vi "Vision Processing Ian.vi"(4 "error in (no error)":errorcluster, 7 "Image Size Gear":T4=enum."160x120") -> ()   [LabVIEW 2016]
doc: "This VI runs in parallel to other tasks. It gets images from the camera, processes them for color or shape and use that information to affect robot behavior."
uses:
  Vision Support Code/Camera Types.ctl
  <vilib>/Rock Robotics/WPI/Camera/WPI_CameraImageSize.ctl
  <vilib>/vision/Measure.llb/Edge Options.ctl
  <vilib>/vision/Measure.llb/Edge Polarity.ctl
  <vilib>/Rock Robotics/WPI/Camera/WPI_CameraExposure Values.ctl
  <vilib>/Rock Robotics/WPI/Camera/WPI_CameraWhite Balance Values.ctl
  <vilib>/Rock Robotics/WPI/Camera/WPI_CameraFrameRate.ctl
  <vilib>/vision/NI_Vision_Development_Module.lvlib
panel:
  in  "Edge Options Gear":T1={"Edge Polarity"=0, "Kernel Size"=3, "Width"=3, "Minimum Edge Strength"=18.0, "Interpolation Type"=enum."Bilinear Fixed", "Data Processing Method"=enum."Average"} {"Edge Polarity" items=["All Edges", "Rising Edges", "Falling Edges"]; "Minimum Edge Strength" format="%.2f"; "Width" step=2; "Kernel Size" step=2}
  in  "boresight":dbl=24.9
  in  "Factor to Distance":dbl=12.0
  in  "Ball?":bool=TRUE
  in  "LED Color Ball":T3={"Hue"={189.50518161930526, 233.66474196477665}, "Sat"={33.39285714285715, 185.17857142857144}, "Val"={15.178571428571438, 255.0}} {"Hue" scale=0.0..255.0 scale format="%#_3g"}
  in  "Brightness":i32=30
  in  "Exposure (%)":dbl format="%#_13g"
  in  "Color Temp (K)":dbl=4000.0 format="%#_13g"
  in  "Edge Options":T1={"Edge Polarity"=0, "Kernel Size"=3, "Width"=3, "Minimum Edge Strength"=2.0, "Interpolation Type"=enum."Bilinear Fixed", "Data Processing Method"=enum."Average"} {"Edge Polarity" items=["All Edges", "Rising Edges", "Falling Edges"]; "Minimum Edge Strength" format="%.2f"; "Width" step=2; "Kernel Size" step=2}
  in  "Size Limit %":dbl=0.04 format="%#_13g"
  in  "Cal Turret":bool
  out "Calibration error 2":errorcluster={"status"=TRUE, "code"=-1074396074, "source"=""}
  out "Physical Paths":string[](array[string])=["-0_1_1_1_0", "-0_1_2_1_0"]
  out "Logical Paths":string[](array[string])=["video0", "video1"]
  out "Gear Valid":bool
  out "Boiler Yaw Delta":dbl=-17.15
  out "Boiler Valid":bool
  out "Boiler Distance":dbl=inf
  in  "Angle":enum16{"Horizontal", "Vertical", "Diagonal"}(ring)=enum."Vertical"
  in  "Gear?":bool=TRUE
  in  "Image SizeTurr":T4=enum."160x120"
  in  "Score Cutoff Turret":dbl=70.0
  out "Gear Distance":dbl=inf
  out "Gear Yaw Delta":dbl=-5.600000000000001
  in  "FOV":cluster{"X (degrees)":dbl, "Y (degrees)":dbl}={"X (degrees)"=34.3, "Y (degrees)"=61.0}
  in  "Height":T5={"Hc (GND to lense)"=12.5, "Ht (GND to CTR)"=0.0}
  in  "LED Color Target":T3={"Hue"={217.1650671807445, 7.296259223023774}, "Sat"={115.35714285714286, 255.0}, "Val"={21.25000000000001, 255.0}} {"Hue" scale=0.0..255.0 scale format="%#_3g"}
  in  "Camera Type":T6=enum."1013"
  in  "Score Cutoff %":dbl=50.0
  in  "Particles":dbl=5.0
  in  "Color Mode":u16(ring)=3 items=["RGB", "HSL", "HSV", "HSI"]
  in  "Use Calibration":bool
  out "Calibration error":errorcluster
  in  "Line Border":cluster{"Top":dbl, "Bottom":dbl}={"Top"=6.0, "Bottom"=1.0}
  in  "Display Original":bool=TRUE
  in  "Display Mask":bool=TRUE
  out "Mask":T7(plugin-control)
  out "Original Image":T7(plugin-control)
  out "loop ms":u32=117
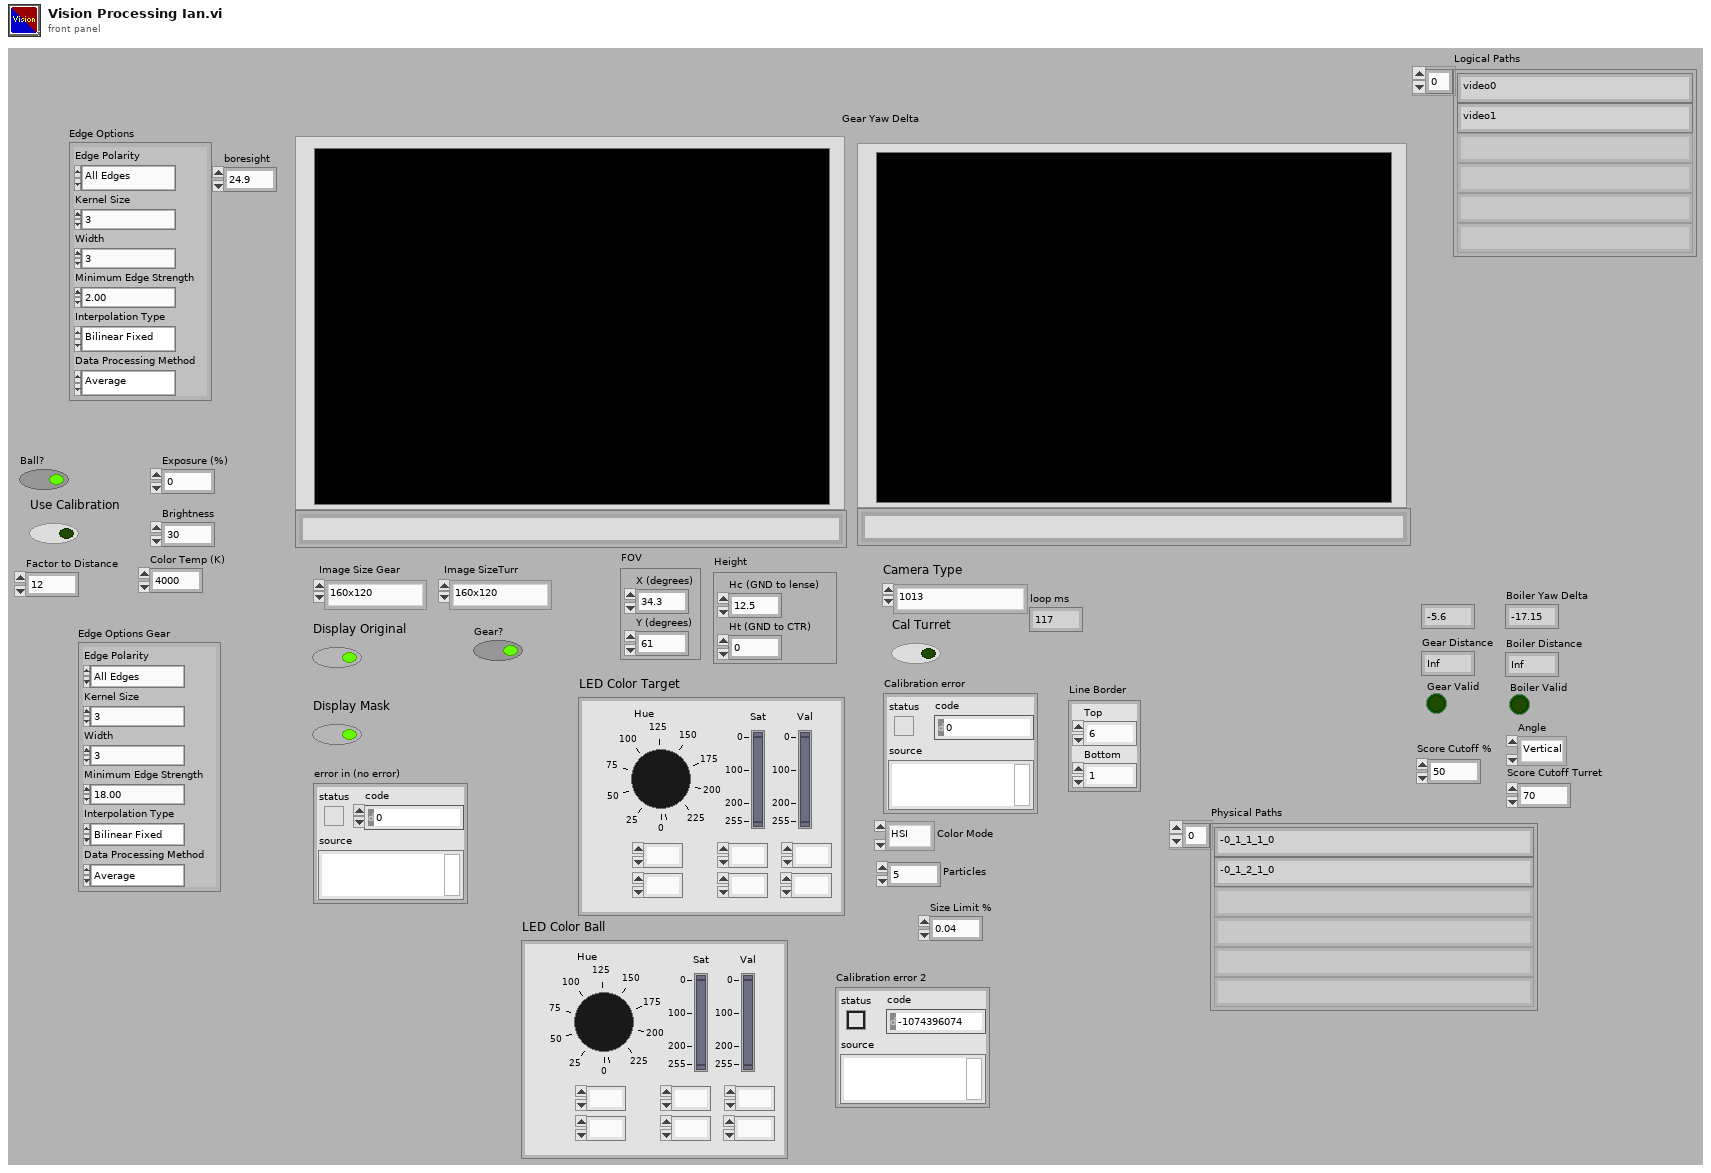
[diagram p1: front panel]
types:
  T1 = typedef "Edge Options.ctl" = cluster{"Edge Polarity":T2, "Kernel Size":u32, "Width":u32, "Minimum Edge Strength":sgl, "Interpolation Type":enum32{"Zero Order", "Bilinear", "Quadratic", "Cubic", "Bilinear Fixed"}, "Data Processing Method":enum32{"Average", "Median"}}
  T2 = typedef "Edge Polarity.ctl" = u32
  T3 = cluster{"Hue":cluster{dbl, dbl}, "Sat":cluster{dbl, dbl}, "Val":cluster{dbl, dbl}}
  T4 = typedef "WPI_CameraImageSize.ctl" = enum16{"640x480", "320x240", "160x120", "Custom"}
  T5 = cluster{"Hc (GND to lense)":dbl, "Ht (GND to CTR)":dbl}
  T6 = typedef "Camera Types.ctl" = enum16{"206", "1011", "1013", "MS HD3000 square", "MS HD3000 640x480"}
  T7 = typedef "IMAQ Image.ctl" = refnum<image>
  T8 = typedef "Image Type" = u32
  T9 = typedef "WPI_CameraFrameRate.ctl" = u32
  T10 = typedef "WPI_CameraExposure Values.ctl" = enum16{"Auto", "Flicker-free 50 Hz", "Flicker-free 60 Hz", "Hold current", "Custom"}
  T11 = typedef "WPI_CameraWhite Balance Values.ctl" = enum16{"Auto", "Fixed indoor", "Fixed outdoor 1", "Fixed outdoor 2", "Fixed fluorescent 1", "Fixed fluorescent 2", "Hold current", "Custom"}
  T12 = typedef "Particle Parameters" = i32
  T13 = typedef "WPI_CameraDevRef.ctl" = cluster{"Camera Address":string, "CameraStatus":errorcluster}
  T14 = cluster{"Left":dbl, "Top":dbl, "Right":dbl, "Bottom":dbl}
  T15 = cluster{"Distance (ft)":dbl, "Score":dbl, "Normalized":cluster{"Center":cluster{dbl, dbl}, "Rectangle":cluster{"Numeric":dbl, "Numeric 2":dbl, "Numeric 3":dbl, "Numeric 5":dbl}}, "Pixels":cluster{"Center":cluster{dbl, dbl}, "Rectangle":cluster{"Numeric":dbl, "Numeric 2":dbl, "Numeric 3":dbl, "Numeric 5":dbl}}}
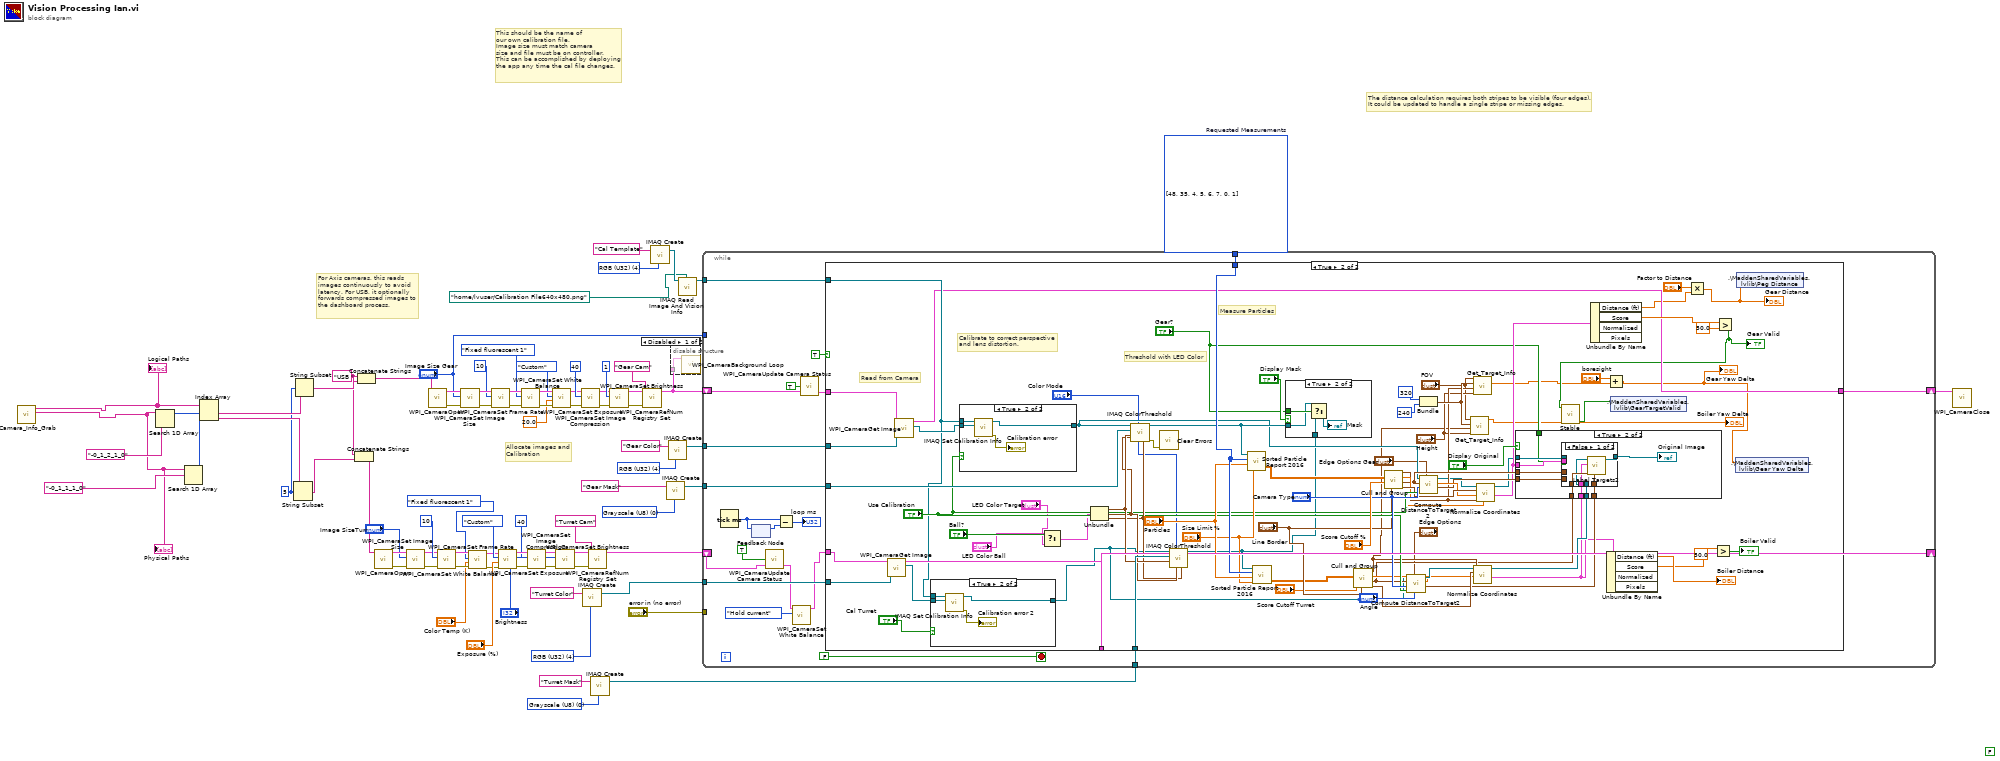
[diagram p0: block diagram]
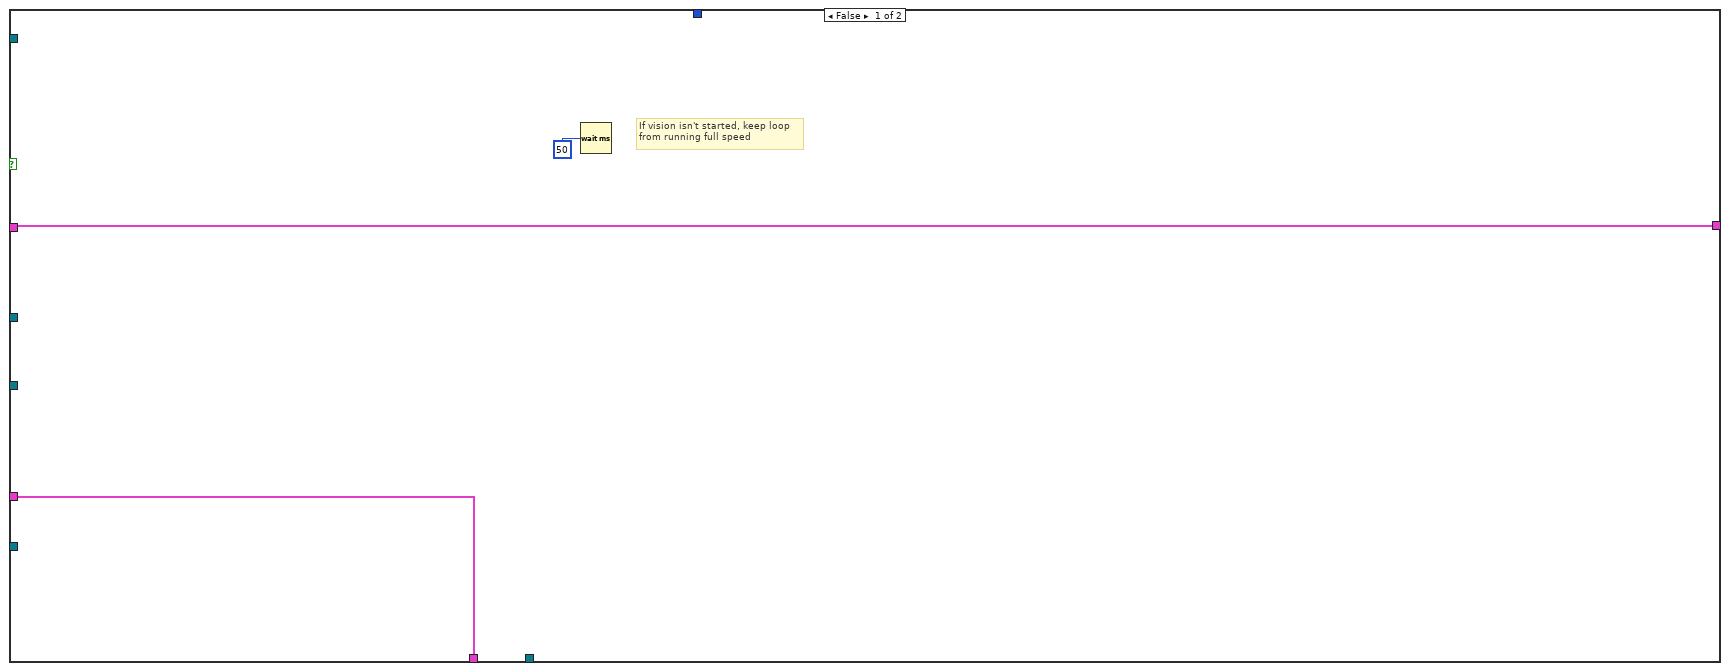
[diagram p3: hidden frame]
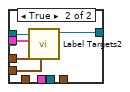
[diagram p6: hidden frame]
diagram:
  (unwired) FALSE
  w14 = "USB " ("string")
  w16 = 5 ("offset (0)")
  w24 = T8 0 items=["Grayscale (U8)", "Grayscale (I16)", "Grayscale (SGL)", "Complex (CSG)", "RGB (U32)", "HSL (U32)", "RGB (U64)", "Grayscale (U16)"] ("Image Type")
  w26 = T8 4 items=["Grayscale (U8)", "Grayscale (I16)", "Grayscale (SGL)", "Complex (CSG)", "RGB (U32)", "HSL (U32)", "RGB (U64)", "Grayscale (U16)"] ("Image Type")
  w74 = T8 4 items=["Grayscale (U8)", "Grayscale (I16)", "Grayscale (SGL)", "Complex (CSG)", "RGB (U32)", "HSL (U32)", "RGB (U64)", "Grayscale (U16)"] ("Image Type")
  w79 = T8 0 items=["Grayscale (U8)", "Grayscale (I16)", "Grayscale (SGL)", "Complex (CSG)", "RGB (U32)", "HSL (U32)", "RGB (U64)", "Grayscale (U16)"] ("Image Type")
  w80 = T8 4 items=["Grayscale (U8)", "Grayscale (I16)", "Grayscale (SGL)", "Complex (CSG)", "RGB (U32)", "HSL (U32)", "RGB (U64)", "Grayscale (U16)"] ("Image Type")
  w76 = T12[] [48, 35, 4, 5, 6, 7, 0, 1] items=["Center of Mass X", "Center of Mass Y", "First Pixel X", "First Pixel Y", "Bounding Rect Left", "Bounding Rect Top", "Bounding Rect Right", "Bounding Rect Bottom", "Max Feret Diameter Start X", "Max Feret Diameter Start Y", "Max Feret Diameter End X", "Max Feret Diameter End Y", "Max Horiz. Segment Length Left", "Max Horiz. Segment Length Right", "Max Horiz. Segment Length Row", "-", "Bounding Rect Width", "Bounding Rect Height", "Bounding Rect Diagonal", "Perimeter", "Convex Hull Perimeter", "Holes' Perimeter", "Max Feret Diameter", "Equivalent Ellipse Major Axis", "Equivalent Ellipse Minor Axis", "Equivalent Ellipse Minor Axis (Feret)", "Equivalent Rect Long Side", "Equivalent Rect Short Side", "Equivalent Rect Diagonal", "Equivalent Rect Short Side (Feret)", "Average Horiz. Segment Length", "Average Vert. Segment Length", "Hydraulic Radius", "Waddel Disk Diameter", "-", "Area", "Holes' Area", "Particle & Holes' Area", "Convex Hull Area", "Image Area", "-", "Number of Holes", "Number of Horiz. Segments", "Number of Vert. Segments", "-", "Orientation", "Max Feret Diameter Orientation", "-", "% Area/Image Area", "% Area/(Particle & Holes' Area)", "Ratio of Equivalent Ellipse Axes", "Ratio of Equivalent Rect Sides", "-", "Elongation Factor", "Compactness Factor", "Heywood Circularity Factor", "Type Factor", "-", "Sum X", "Sum Y", "Sum XX", "Sum XY", "Sum YY", "Sum XXX", "Sum XXY", "Sum XYY", "Sum YYY", "-", "Moment of Inertia XX", "Moment of Inertia XY", "Moment of Inertia YY", "Moment of Inertia XXX", "Moment of Inertia XXY", "Moment of Inertia XYY", "Moment of Inertia YYY", "Norm. Moment of Inertia XX", "Norm. Moment of Inertia XY", "Norm. Moment of Inertia YY", "Norm. Moment of Inertia XXX", "Norm. Moment of Inertia XXY", "Norm. Moment of Inertia XYY", "Norm. Moment of Inertia YYY", "Hu Moment 1", "Hu Moment 2", "Hu Moment 3", "Hu Moment 4", "Hu Moment 5", "Hu Moment 6", "Hu Moment 7"]  # Requested Measurements
  # "For Axis cameras, this reads\nimages continuously to avoid\nlatency. For USB, it optionally\nforwards compressed images to\nthe dashboard process."
  # "Allocate images and\nCalibration"
  # "This should be the name of \nour own calibration file.\nImage size must match camera\nsize and file must be on controller.\nThis can be accomplished by deploying\nthe app any time the cal file changes."
  # "The distance calculation requires both stripes to be visible (four edges).\nIt could be updated to handle a single stripe or missing edges."
  n1 = call <userlib>:"Camera_Info_Grab.vi"() -> ("Physical Paths"=w8:string[], "Logical Paths"=w9:string[])  [unwired: 10 in]
  "Logical Paths" <- w9
  "Physical Paths" <- w8
  n2 = Search 1D Array(1D array=w8, element="-0_1_2_1_0") -> (index of element=w20:i32)  [unwired: 1 in]
  n3 = Search 1D Array(1D array=w8, element="-0_1_1_1_0") -> (index of element=w19:i32)  [unwired: 1 in]
  n4 = Index Array(array=w9, index #1=w20, index #2=w19) -> (element #1=w18:string, element #2=w17:string)
  n5 = String Subset(string=w17, offset (0)=w16) -> (substring=w13:string)  [unwired: 1 in]
  n6 = String Subset(string=w18, offset (0)=w16) -> (substring=w15:string)  [unwired: 1 in]
  n7 = Concatenate Strings(w14, w13) -> (w12:string)
  n8 = Concatenate Strings(w14, w15) -> (w11:string)
  n9 = call <vilib>:"WPI_CameraOpen.vi"("Camera Address"=w12) -> ("error out"=w39:errorcluster, "CameraDevRef"=w38:T13)  [unwired: 1 in, 8 out]
  n10 = call <vilib>:"WPI_CameraSet Image Size.vi"("error in (no error)"=w39, "Image Size"="Image SizeTurr", "CameraDevRef"=w38) -> ("error out"=w40:errorcluster, "CameraDevRef Out"=w37:T13)  [unwired: 1 in, 6 out]
  n11 = call <vilib>:"WPI_CameraOpen.vi"("Camera Address"=w11) -> ("error out"=w60:errorcluster, "CameraDevRef"=w61:T13)  [unwired: 1 in, 8 out]
  n12 = call <vilib>:"WPI_CameraSet Frame Rate.vi"("error in (no error)"=w40, "Frame Rate (fps)"=T9 10, "CameraDevRef"=w37) -> ("error out"=w4:errorcluster, "CameraDevRef Out"=w6:T13)  [unwired: 7 out]
  n13 = call <vilib>:"WPI_CameraSet Image Size.vi"("error in (no error)"=w60, "Image Size"="Image Size Gear", "CameraDevRef"=w61) -> ("error out"=w59:errorcluster, "CameraDevRef Out"=w62:T13)  [unwired: 1 in, 6 out]
  n14 = call <vilib>:"WPI_CameraSet White Balance.vi"("error in (no error)"=w4, "Color Temp (K)"="Color Temp (K)", "White Balance"=WPI_CameraWhite_Balance_Values."Fixed fluorescent 1", "CameraDevRef"=w6) -> ("error out"=w3:errorcluster, "CameraDevRef Out"=w5:T13)  [unwired: 6 in]
  n15 = call <vilib>:"WPI_CameraSet Frame Rate.vi"("error in (no error)"=w59, "Frame Rate (fps)"=T9 10, "CameraDevRef"=w62) -> ("error out"=w58:errorcluster, "CameraDevRef Out"=w64:T13)  [unwired: 7 out]
  n16 = call <vilib>:"WPI_CameraSet Exposure.vi"("error in (no error)"=w3, "Exposure (%)"="Exposure (%)", "Exposure"=WPI_CameraExposure_Values."Custom", "CameraDevRef"=w5) -> ("error out"=w41:errorcluster, "CameraDevRef Out"=w35:T13)  [unwired: 6 out]
  n17 = call <vilib>:"WPI_CameraSet White Balance.vi"("error in (no error)"=w58, "White Balance"=WPI_CameraWhite_Balance_Values."Fixed fluorescent 1", "CameraDevRef"=w64) -> ("error out"=w57:errorcluster, "CameraDevRef Out"=w63:T13)  [unwired: 1 in, 6 out]
  n18 = call <vilib>:"WPI_CameraSet Image Compression.vi"("error in (no error)"=w41, "Compression"=40, "CameraDevRef"=w35) -> ("error out"=w42:errorcluster, "CameraDevRef Out"=w36:T13)  [unwired: 7 out]
  n19 = call <vilib>:"WPI_CameraSet Exposure.vi"("error in (no error)"=w57, "Exposure (%)"=20.0, "Exposure"=WPI_CameraExposure_Values."Custom", "CameraDevRef"=w63) -> ("error out"=w56:errorcluster, "CameraDevRef Out"=w66:T13)  [unwired: 6 out]
  n20 = call <vilib>:"WPI_CameraSet Brightness.vi"("error in (no error)"=w42, "Brightness"="Brightness", "CameraDevRef"=w36) -> ("error out"=w43:errorcluster, "CameraDevRef Out"=w30:T13)  [unwired: 7 out]
  n21 = call <vilib>:"WPI_CameraSet Image Compression.vi"("error in (no error)"=w56, "Compression"=40, "CameraDevRef"=w66) -> ("error out"=w55:errorcluster, "CameraDevRef Out"=w65:T13)  [unwired: 7 out]
  n22 = call "IMAQ Create"("Image Name"="Turret Color", "Image Type"=w26) -> ("New Image"=w25:T7)  [unwired: 2 in, 2 out]
  n23 = call <vilib>:"WPI_CameraRefNum Registry Set.vi"("error in (no error)"=w43, "refnum name"="Turret Cam", "CameraDevRef"=w30) -> ("CameraDevRef"=w28:T13)  [unwired: 1 in, 7 out]
  n24 = call "IMAQ Create"("Image Name"="Turret Mask", "Image Type"=w24) -> ("New Image"=w22:T7)  [unwired: 2 in, 2 out]
  n25 = call <vilib>:"WPI_CameraSet Brightness.vi"("error in (no error)"=w55, "Brightness"=1, "CameraDevRef"=w65) -> ("error out"=w54:errorcluster, "CameraDevRef Out"=w70:T13)  [unwired: 7 out]
  n26 = call <vilib>:"WPI_CameraRefNum Registry Set.vi"("error in (no error)"=w54, "refnum name"="Gear Cam", "CameraDevRef"=w70) -> ("CameraDevRef"=w50:T13)  [unwired: 1 in, 7 out]
  n27 = call "IMAQ Create"("Image Name"="Cal Template", "Image Type"=w74) -> ("New Image"=w72:T7)  [unwired: 2 in, 2 out]
  n28 = call "IMAQ Create"("Image Name"="Gear Mask", "Image Type"=w79) -> ("New Image"=w77:T7)  [unwired: 2 in, 2 out]
  n29 = call "IMAQ Create"("Image Name"="Gear Color", "Image Type"=w80) -> ("New Image"=w75:T7)  [unwired: 2 in, 2 out]
  n30 = disable-structure shown="Disabled" {
    disable-tunnel: w50 -> [w82 _]
    frame Disabled {
      n31 = call <vilib>:"WPI_CameraBackground Loop.vi"("CameraDevRef"=w82) -> ()  [unwired: 11 in]
    }
    frame Enabled {
    }
  }
  n32 = call "IMAQ Read Image And Vision Info"("File Path"=path "/home/lvuser/Calibration File640x480.png" ("Folder Location"), "Image"=w72) -> ("Image Out"=w71:T7)  [unwired: 7 in, 2 out]
  n33 = while {
    tunnel: w75 -> [w99]
    tunnel: w77 -> [w102]
    tunnel: w76 -> [w101]
    tunnel: w71 -> [w100]
    shift-right: [w98] -> w49
    shift-left: w50 -> [w97]
    tunnel: "error in (no error)" -> [_]
    tunnel: "Image Size Gear" -> [_]
    shift-right: [w92] -> _
    shift-left: w28 -> [w87]
    tunnel: w25 -> [w91]
    tunnel: w22 -> [w90]
    stop <- FALSE ("Boolean") stop-if-true
    n34 = Tick Count (ms)() -> (millisecond timer value=w94:u32)
    n35 = feedback-in #1(w94) -> ()
    n36 = feedback #1() -> (w95:u32)  [unwired: 1 in]
    n37 = call <vilib>:"WPI_CameraUpdate Camera Status.vi"("CameraDevRef In"=w87, "Enable Vision"=TRUE) -> ("CameraDevRef Out"=w85:T13)  [unwired: 3 in]
    n38 = Subtract(x=w94, y=w95) -> (x-y=→"loop ms":u32)
    n39 = call <vilib>:"WPI_CameraSet White Balance.vi"("White Balance"=WPI_CameraWhite_Balance_Values."Hold current", "CameraDevRef"=w85) -> ("CameraDevRef Out"=w84:T13)  [unwired: 8 in, 1 out]
    n40 = call <vilib>:"WPI_CameraUpdate Camera Status.vi"("CameraDevRef In"=w97, "Enable Vision"=TRUE) -> ("CameraDevRef Out"=w96:T13)  [unwired: 3 in]
    n41 = case shown="True" TRUE {
      tunnel: w102 -> [_ w185]
      tunnel: w101 -> [_ w174]
      tunnel: w100 -> [_ w125]
      tunnel: w96 -> [w106 w184]
      tunnel: w99 -> [_ w179]
      tunnel: [w106 w120] -> w98
      tunnel: w84 -> [w104 w182]
      tunnel: [w104 w181] -> w92
      tunnel: w91 -> [_ w180]
      tunnel: w90 -> [_ w178]
      frame False {
        # "If vision isn't started, keep loop\nfrom running full speed"
        n42 = Wait (ms)(milliseconds to wait=u32 50) -> ()  [unwired: 1 out]
      }
      frame True {
        # "Read from Camera"
        # "Calibrate to correct perspective\nand lens distortion."
        # "Measure Particles"
        # "Threshold with LED Color"
        n43 = call <vilib>:"WPI_CameraGet Image.vi"("Image"=w180, "CameraDevRef"=w182) -> ("Image Out"=w124:T7, "CameraDevRef Out"=w181:T13)  [unwired: 7 in, 1 out]
        n44 = call <vilib>:"WPI_CameraGet Image.vi"("Image"=w179, "CameraDevRef"=w184) -> ("Image Out"=w137:T7, "CameraDevRef Out"=w120:T13)  [unwired: 7 in, 1 out]
        n45 = case shown="True" "Cal Turret" {
          tunnel: [w186 w190] -> w123
          tunnel: w124 -> [w186 w189]
          tunnel: w125 -> [_ w188]
          frame False {
          }
          frame True {
            n46 = call "IMAQ Set Calibration Info"("Image Dst"=w189, "Image Src"=w188) -> ("error out"=→"Calibration error 2":errorcluster, "Calibrated Image"=w190:T7)  [unwired: 8 in]
          }
        }
        n47 = case shown="True" "Use Calibration" {
          tunnel: [w215 w219] -> w145
          tunnel: w137 -> [w215 w218]
          tunnel: w125 -> [_ w217]
          frame False {
          }
          frame True {
            n48 = call "IMAQ Set Calibration Info"("Image Dst"=w218, "Image Src"=w217) -> ("error out"=→"Calibration error":errorcluster, "Calibrated Image"=w219:T7)  [unwired: 8 in]
          }
        }
        n49 = Select(t="LED Color Ball", s="Ball?", f="LED Color Target") -> (s? t:f=w116:T3)
        n50 = Unbundle(w116) -> ("Hue"=w177:cluster{dbl, dbl}, "Sat"=w176:cluster{dbl, dbl}, "Val"=w175:cluster{dbl, dbl})
        n51 = call "IMAQ ColorThreshold"("Blue or Luma or Val or Inten Range"=w175, "Green or Sat Range"=w176, "Color Mode"="Color Mode", "Red or Hue Range"=w177, "Image Dst"=w185, "Image Src"=w145) -> ("error out"=w157:errorcluster, "Image Dst Out"=w156:T7)  [unwired: 4 in]
        n52 = call <vilib>:"Clear Errors.vi"("error in (no error)"=w157) -> ()  [unwired: 5 in, 2 out]
        n53 = call "IMAQ ColorThreshold"("Blue or Luma or Val or Inten Range"=w175, "Green or Sat Range"=w176, "Color Mode"="Color Mode", "Red or Hue Range"=w177, "Image Dst"=w178, "Image Src"=w123) -> ("Image Dst Out"=w132:T7)  [unwired: 4 in, 1 out]
        n54 = call "Sorted Particle Report 2016.vi"("Min Area Size %"="Size Limit %", "Particle Count Limit"="Particles", "Pixel Measurements"=w174, "Image in"=w156) -> ("Sorted Data"=w146:dbl[][])  [unwired: 1 out]
        n55 = call "Sorted Particle Report 2016.vi"("Min Area Size %"="Size Limit %", "Particle Count Limit"="Particles", "Pixel Measurements"=w174, "Image in"=w132) -> ("Sorted Data"=w167:dbl[][])  [unwired: 1 out]
        n56 = case shown="True" "Display Mask" {
          tunnel: w156 -> [_ w212]
          tunnel: "Gear?" -> [_ w214]
          tunnel: w132 -> [_ w211]
          frame False {
          }
          frame True {
            n57 = Select(t=w212, s=w214, f=w211) -> (s? t:f=→"Mask":T7)
          }
        }
        n58 = call "Cull and Group.vi"("Line Border"="Line Border", "Score Cutoff"="Score Cutoff Turret", "Sorted Data"=w167) -> ("Rect"=w164:T14, "Line"=w130:T14, "Score"=w163:dbl, "Center"=w131:cluster{"X":dbl, "Y":dbl})  [unwired: 5 in]
        n59 = call "Cull and Group.vi"("Line Border"="Line Border", "Score Cutoff"="Score Cutoff %", "Sorted Data"=w146) -> ("Rect"=w155:T14, "Line"=w152:T14, "Score"=w153:dbl, "Center"=w143:cluster{"X":dbl, "Y":dbl})  [unwired: 5 in]
        n60 = call "Compute DistanceToTarget2.vi"("Angle"="Angle", "Edge Options"="Edge Options", "Calibrated"="Use Calibration", "Camera Type"="Camera Type", "Line"=w130, "Image Src"=w123) -> ("Edges"=w129:cluster{"X":sgl, "Y":sgl}[], "Distance (ft)"=w162:dbl, "Image Dst Out"=w165:T7)  [unwired: 3 in]
        n61 = Bundle(320, 240) -> (w144:cluster{i32, i32})  [unwired: 1 in]
        n62 = call "Compute DistanceToTarget2.vi"("Edge Options"="Edge Options Gear", "Calibrated"="Use Calibration", "Camera Type"="Camera Type", "Line"=w152, "Image Src"=w145) -> ("Edges"=w151:cluster{"X":sgl, "Y":sgl}[], "Distance (ft)"=w154:dbl, "Image Dst Out"=w140:T7)  [unwired: 4 in]
        n63 = call "Get_Target_Info.vi"("Height"="Height", "Target Location"=w131, "Resolution"=w144, "FOV"="FOV") -> ("Yaw Delta"=→"Boiler Yaw Delta":dbl)  [unwired: 4 in, 3 out]
        n64 = call "Get_Target_Info.vi"("Height"="Height", "Target Location"=w143, "Resolution"=w144, "FOV"="FOV") -> ("Elevation Delta"=w107:dbl)  [unwired: 4 in, 3 out]
        n65 = call "Normalize Coordinates.vi"("Score"=w163, "Center"=w131, "Distance"=w162, "Bounding box"=w164, "Image in"=w165) -> ("Results"=w127:T15, "Image out"=w128:T7)  [unwired: 5 in]
        n66 = call "Normalize Coordinates.vi"("Score"=w153, "Center"=w143, "Distance"=w154, "Bounding box"=w155, "Image in"=w140) -> ("Results"=w148:T15, "Image out"=w147:T7)  [unwired: 5 in]
        n67 = case shown="True" "Display Original" {
          tunnel: w147 -> [_ w199]
          tunnel: w148 -> [_ w198]
          tunnel: w152 -> [_ w197]
          tunnel: w151 -> [_ w196]
          tunnel: "Gear?" -> [_ w195]
          tunnel: w130 -> [_ w194]
          tunnel: w129 -> [_ w193]
          tunnel: w128 -> [_ w192]
          tunnel: w127 -> [_ w191]
          frame False {
          }
          frame True {
            n68 = case shown="False" w195 {
              tunnel: [w205 w210] -> w200
              tunnel: w199 -> [_ w209]
              tunnel: w198 -> [_ w208]
              tunnel: w197 -> [_ w207]
              tunnel: w196 -> [_ w206]
              tunnel: w194 -> [w204 _]
              tunnel: w193 -> [w203 _]
              tunnel: w192 -> [w202 _]
              tunnel: w191 -> [w201 _]
              frame False {
                n69 = call "Label Targets2.vi"("Edges"=w203, "Line"=w204, "Results"=w201, "Image in"=w202) -> ("Image out"=w205:T7)  [unwired: 7 in]
              }
              frame True {
                n70 = call "Label Targets2.vi"("Edges"=w206, "Line"=w207, "Results"=w208, "Image in"=w209) -> ("Image out"=w210:T7)  [unwired: 7 in]
              }
            }
            "Original Image" <- w200
          }
        }
        n71 = Unbundle By Name(w148) -> ("Distance (ft)"=w113:dbl, "Score"=w136:dbl)  [unwired: 2 out]
        n72 = Unbundle By Name(w127) -> ("Distance (ft)"=→"Boiler Distance":dbl, "Score"=w160:dbl)  [unwired: 2 out]
        n73 = Add(x="boresight", y=w107) -> (x+y=w112:dbl)
        "Gear Yaw Delta" <- w112
        n74 = Multiply(x="Factor to Distance", y=w113) -> (x*y=w115:dbl)
        "Gear Distance" <- w115
        n75 = Greater?(x=w160, y=50.0) -> (0:→"Boiler Valid":bool)
        n76 = Greater?(x=w136, y=50.0) -> (0:w110:bool)
        "Gear Valid" <- w110
        n77 = call <userlib>:"Stable.vi"("Signal Input"=w110) -> ("Stable"=w109:bool)  [unwired: 10 in]
        n78 = shared-variable ".\\MaddenSharedVariables.lvlib\\GearTargetValid"(w109) -> ()  [unwired: 1 in, 1 out]
        n79 = shared-variable ".\\MaddenSharedVariables.lvlib\\Gear Yaw Delta"(w112) -> ()  [unwired: 1 in, 1 out]
        n80 = shared-variable ".\\MaddenSharedVariables.lvlib\\Peg Distance"(w115) -> ()  [unwired: 1 in, 1 out]
      }
    }
  }
  n81 = call <vilib>:"WPI_CameraClose.vi"("CameraDevRef"=w49) -> ()  [unwired: 1 in, 10 out]
